vi "URL.vi"(8 "比例尺":dbl, 10 "纬度":dbl, 11 "经度":dbl) -> (2 "URL":string)   [LabVIEW 2018]
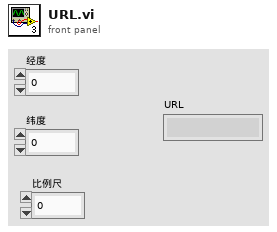
[diagram p1: front panel]
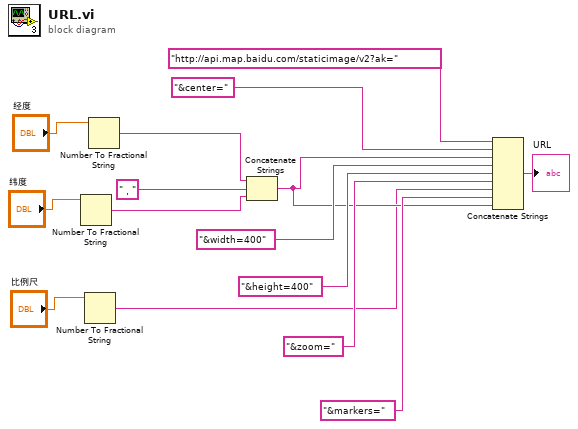
[diagram p0: block diagram]
diagram:
  n1 = Number To Fractional String(number="纬度") -> (F-format string=w3:string)  [unwired: 3 in]
  n2 = Number To Fractional String(number="比例尺") -> (F-format string=w1:string)  [unwired: 3 in]
  n3 = Number To Fractional String(number="经度") -> (F-format string=w5:string)  [unwired: 3 in]
  n4 = Concatenate Strings(w5, "，", w3) -> (w8:string)
  n5 = Concatenate Strings("http://api.map.baidu.com/staticimage/v2?ak=", "&center=", w8, "&width=400", "&height=400", "&zoom=", w1, "&markers=", w8) -> (→"URL":string)
